vi "Delay Vec.vi"(2 "initialize":bool, 3 "Delay length":i32, 5 "X":sgl[](array[numeric])=[0.0] format="%0.2f") -> (1 "Delayed X":sgl[](array[numeric]) format="%0.2f")   [LabVIEW 2013]
panel:
  # "Delay a multi-channel signal for an integral number of cycles, >=1"
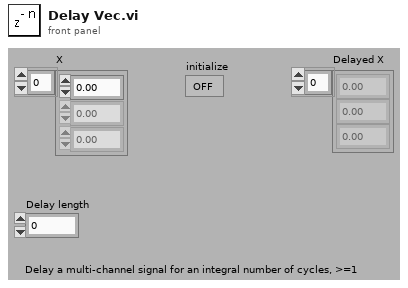
[diagram p1: front panel]
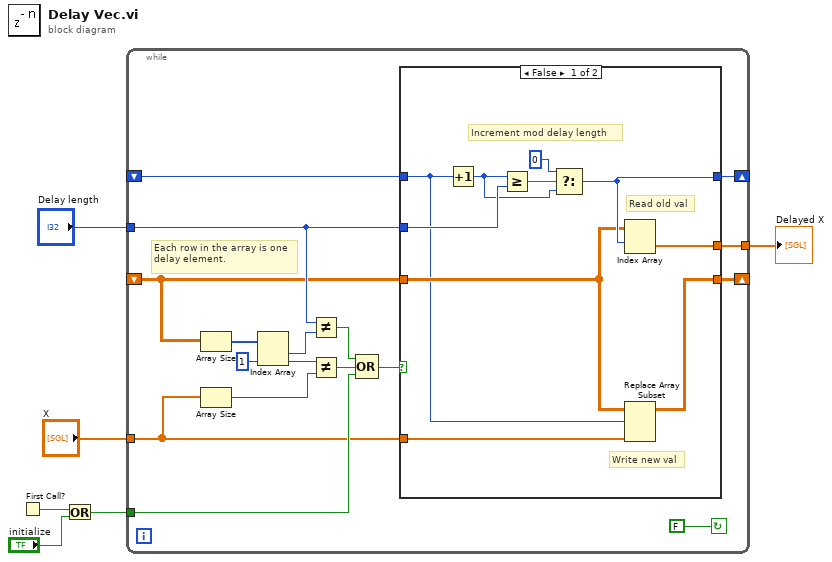
[diagram p0: block diagram]
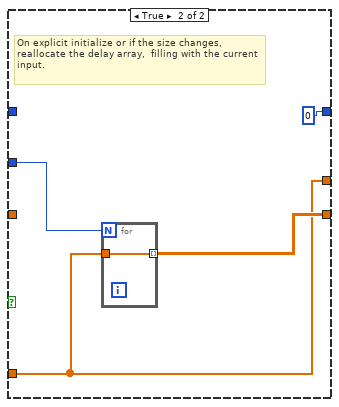
[diagram p2: hidden frame]
diagram:
  n1 = First Call?() -> (First Call?: T/F=w3:bool)
  n2 = Or(x=w3, y="initialize") -> (x .or. y?=w5:bool)
  n3 = while {
    tunnel: "X" -> [w12]
    tunnel: w5 -> [w15]
    shift-right: [w11] -> _
    shift-left: _ -> [w9]
    tunnel: "Delay length" -> [w13]
    shift-right: [w10] -> _
    shift-left: _ -> [w8]
    tunnel: [w7] -> w1
    stop <- FALSE continue-if-true
    # "Each row in the array is one delay element."
    n4 = Array Size(array=w9) -> (size(s)=w22:i32[])
    n5 = Array Size(array=w12) -> (size(s)=w18:i32)
    n6 = Index Array(array=w22, index #2=1 ("index")) -> (element #1=w20:i32, element #2=w19:i32)  [unwired: 1 in]
    n7 = Not Equal?(x=w13, y=w20) -> (x != y?=w16:bool)
    n8 = Not Equal?(x=w19, y=w18) -> (x != y?=w17:bool)
    n9 = Compound Arithmetic op=OR(w16, w17, w15) -> (w14:bool)
    n10 = case shown="False" w14 {
      tunnel: w13 -> [w32 w37]
      tunnel: w12 -> [w25 w34]
      tunnel: [w24 w36] -> w11
      tunnel: [w28 0 ("Delay length")] -> w10
      tunnel: w9 -> [w27 _]
      tunnel: w8 -> [w26 _]
      tunnel: [w33 w34] -> w7
      frame False {
        # "Read old val"
        # "Write new val"
        # "Increment mod delay length"
        n11 = Increment(x=w26) -> (x+1=w29:i32)
        n12 = Greater Or Equal?(x=w29, y=w32) -> (x >= y?=w31:bool)
        n13 = Select(t=0 ("x+1"), s=w31, f=w29) -> (s? t:f=w28:i32)
        n14 = Index Array(array=w27, index (row)=w28) -> (element=w33:sgl[])  [unwired: 1 in]
        n15 = Replace Array Subset(array=w27, new element=w25, index (row)=w26) -> (w24:sgl[][])  [unwired: 1 in]
      }
      frame True {
        # "On explicit initialize or if the size changes, reallocate the delay array,  filling with the current input."
        n16 = for {
          N: w37 -> [_]
          tunnel: w34 -> [w38]
          tunnel: [w38] -> w36 mode=indexing
        }
      }
    }
  }
  "Delayed X" <- w1
